vi "Serial Comms - close serial reference.vi"(8 "error in (no error)":errorcluster, 11 "Serial Comms in":refnum<class "Serial Comms.lvclass">) -> (0 "error out":errorcluster, 3 "Serial Comms out":refnum<class "Serial Comms.lvclass">)   [LabVIEW 2020, in "Generic_Comms.lvlib" / "Serial Comms.lvclass"]
uses:
  Serial Comms.lvclass
  Serial Comms.lvclass/Serial Comms.ctl
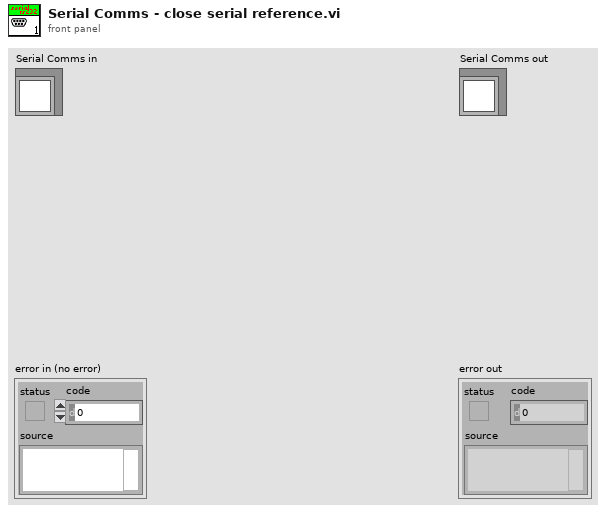
[diagram p1: front panel]
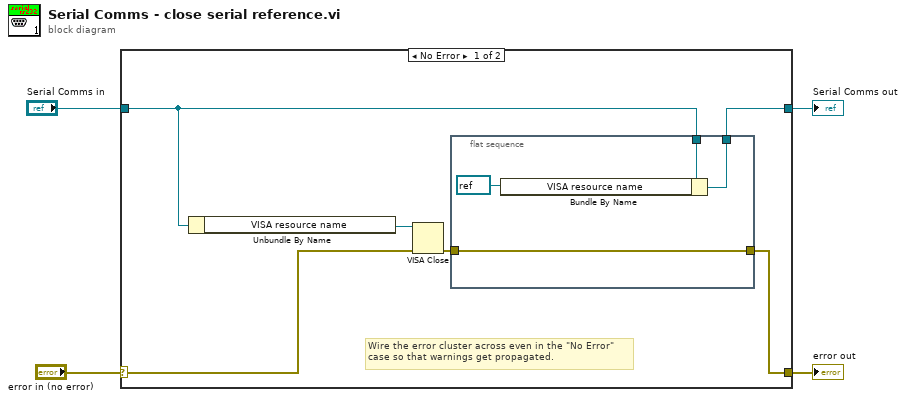
[diagram p0: block diagram]
diagram:
  n1 = case shown="No Error" "error in (no error)" {
    selector: "error in (no error)" -> [w9 w16]
    tunnel: [w5 w16] -> w3
    tunnel: [w7 w15] -> w1
    tunnel: "Serial Comms in" -> [w8 w15]
    frame No Error {
      # "Wire the error cluster across even in the \"No Error\"\ncase so that warnings get propagated."
      n2 = Unbundle By Name(w8) -> ("VISA resource name"=w10:refnum<visa-resource-name>)
      n3 = VISA Close(VISA resource name=w10, error in (no error)=w9) -> (error out=w6:errorcluster)
      n4 = flat-sequence {
        tunnel: w8 -> [w14]
        tunnel: [w12] -> w7
        tunnel: [w11] -> w5
        tunnel: w6 -> [w11]
        frame #0 {
          n5 = Bundle By Name(cluster=w14, "VISA resource name"=refnum<visa-resource-name> refnum) -> (w12:refnum<class "Serial Comms.lvclass">)
        }
      }
    }
    frame Error {
    }
  }
  "error out" <- w3
  "Serial Comms out" <- w1
